vi "Add State to Routing Channel.vi"(8 "error in (no error)":errorcluster, 10 "State and Connections":T1, 11 "Channel Ref in":T3 format="%.0x") -> (0 "error out":errorcluster, 3 "Channel Ref out":T3=18446744073709551615 format="%.0x")   [LabVIEW 2017, in "Routing and Faulting Scripting.lvlib"]
uses:
  Routing and Faulting Scripting.lvlib
  <vilib>/NI Veristand/Custom Device API/Custom Device Item Ref.ctl
  Shared/Routing State.ctl
  Shared/Connection.ctl
  <vilib>/NI VeriStand/Custom Device API/Custom Device API.lvlib
  Shared/Routing and Faulting Shared.lvlib
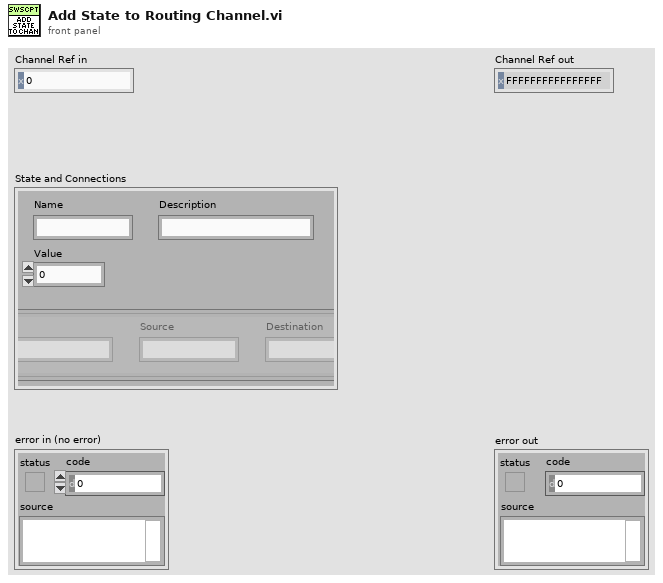
[diagram p1: front panel]
types:
  T1 = typedef "Routing and Faulting Shared.lvlib/Routing State.ctl" = cluster{"Name":string, "Description":string, "Value":i32, "Connection List":T2[]}
  T2 = typedef "Routing and Faulting Shared.lvlib/Connection.ctl" = cluster{"Resource":string, "Source":string, "Destination":string}
  T3 = typedef "Custom Device API.lvlib/Custom Device Item Ref.ctl" = u64
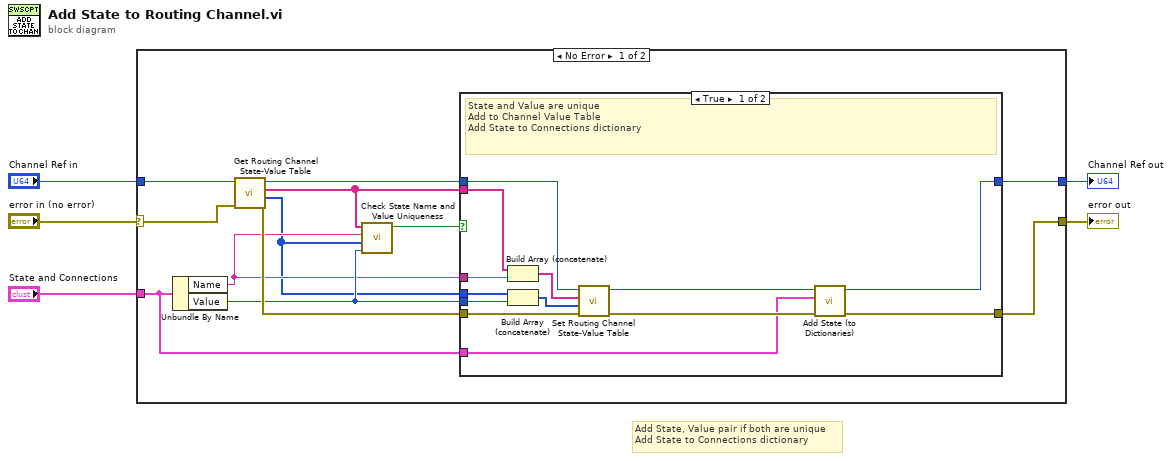
[diagram p0: block diagram]
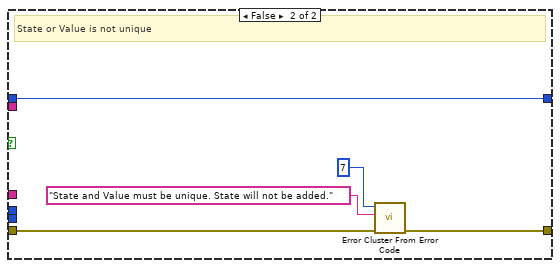
[diagram p2: hidden frame]
diagram:
  # "Add State, Value pair if both are unique\nAdd State to Connections dictionary"
  n1 = case shown="No Error" "error in (no error)" {
    selector: "error in (no error)" -> [w16 w37]
    tunnel: [w12 w37] -> w2
    tunnel: "Channel Ref in" -> [w17 w36]
    tunnel: [w13 w36] -> w3
    tunnel: "State and Connections" -> [w9 _]
    frame No Error {
      n2 = Unbundle By Name(w9) -> ("Name"=w7:string, "Value"=w8:i32)
      n3 = call "Get Routing Channel State-Value Table.vi"("error in (no error)"=w16, "Channel Ref in"=w17) -> ("error out"=w14:errorcluster, "State Values"=w6:i32[], "State Names"=w11:string[], "Channel Ref out"=w15:T3)  [unwired: 6 in]
      n4 = call "Check State Name and Value Uniqueness.vi"("Value"=w8, "State Values"=w6, "Name"=w7, "State Names"=w11) -> ("Is Unique"=w10:bool)  [unwired: 7 in]
      n5 = case shown="True" w10 {
        tunnel: w15 -> [w27 w31]
        tunnel: w14 -> [w26 w33]
        tunnel: w6 -> [w29 _]
        tunnel: [w22 w31] -> w13
        tunnel: [w19 w32] -> w12
        tunnel: w8 -> [w30 _]
        tunnel: w11 -> [w28 _]
        tunnel: w7 -> [w21 _]
        tunnel: w9 -> [w18 _]
        frame True {
          # "State and Value are unique\nAdd to Channel Value Table\nAdd State to Connections dictionary"
          n6 = Build Array (concatenate)(w28, w21) -> (w25:string[])
          n7 = Build Array (concatenate)(w29, w30) -> (w24:i32[])
          n8 = call "Set Routing Channel State-Value Table.vi"("error in (no error)"=w26, "State Values"=w24, "State Names"=w25, "Channel Ref in"=w27) -> ("error out"=w20:errorcluster, "Channel Ref out"=w23:T3)  [unwired: 6 in]
          n9 = call "Add State (to Dictionaries).vi"("error in (no error)"=w20, "Routing Channel State"=w18, "Channel Ref in"=w23) -> ("error out"=w19:errorcluster, "Channel Ref out"=w22:T3)  [unwired: 7 in]
        }
        frame False {
          # "State or Value is not unique"
          n10 = call <vilib>:"Error Cluster From Error Code.vi"("error in (no error)"=w33, "error message (\"\")"="State and Value must be unique. State will not be added." ("error message (\"\")"), "error code (0)"=7) -> ("error out"=w32:errorcluster)  [unwired: 6 in]
        }
      }
    }
    frame Error {
    }
  }
  "Channel Ref out" <- w3
  "error out" <- w2
